vi "SerialOut.vi"(10 "Shutdown Notifier":refnum<notifier>, 11 "Serial Output":refnum<visa-resource-name>="COM6") -> (3 "Done":bool=TRUE)   [LabVIEW 2013]
uses:
  <vilib>/Instr/_visa.llb/VISA Configure Serial Port (Instr).vi
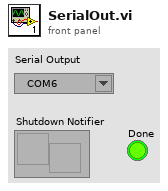
[diagram p1: front panel]
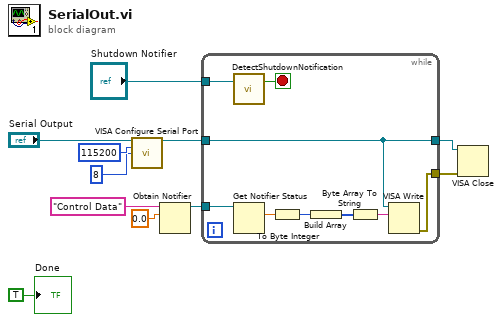
[diagram p0: block diagram]
diagram:
  n1 = call-poly "VISA Configure Serial Port"("VISA resource name"="Serial Output", "baud rate (9600)"=u32 115200, "data bits (8)"=u16 8) -> ("VISA resource name out"=w7:refnum<visa-resource-name>)  [unwired: 11 in, 1 out]
  n2 = Obtain Notifier(name (unnamed)="Control Data", notification data type=0.0 ("number")) -> (notifier out=w1:refnum<notifier>)  [unwired: 2 in, 2 out]
  n3 = while {
    tunnel: [w18] -> w8
    tunnel: w7 -> [w18]
    tunnel: "Shutdown Notifier" -> [w20]
    tunnel: [w17] -> w4
    tunnel: w1 -> [w16]
    stop <- w19 stop-if-true
    n4 = call "DetectShutdownNotification.vi"("Shutdown Notifier"=w20) -> ("Shutdown"=w19:bool)  [unwired: 1 in, 1 out]
    n5 = Get Notifier Status(notifier=w16) -> (current notification=w15:dbl)  [unwired: 1 in, 4 out]
    n6 = To Byte Integer(number=w15) -> (8bit integer=w14:i8)
    n7 = Build Array(w14) -> (w13:i8[])
    n8 = Byte Array To String(unsigned byte array=w13) -> (string=w12:string)
    n9 = VISA Write(VISA resource name=w18, write buffer=w12) -> (error out=w17:errorcluster)  [unwired: 1 in, 2 out]
  }
  n10 = VISA Close(VISA resource name=w8, error in (no error)=w4) -> ()  [unwired: 1 out]
  "Done" <- TRUE
